vi "Kikusui PLZ-Query Error.vi"(8 "error in":errorcluster, 11 "Kikusui PLZ Setting In":T1={"VISA Resource Name"="", "Baud Rate"=19200, "Stop Bits"=20, "Wait For Read(ms)"=0} {"Stop Bits" items=["1.0"=10, "2.0"=20]; "Baud Rate" items=["2400"=2400, "4800"=4800, "9600"=9600, "19200"=19200]}) -> (0 "error out":errorcluster, 3 "Kikusui PLZ Setting Out":T1={"VISA Resource Name"="", "Baud Rate"=19200, "Stop Bits"=20, "Wait For Read(ms)"=0} {"Stop Bits" items=["1.0"=10, "2.0"=20]; "Baud Rate" items=["2400"=2400, "4800"=4800, "9600"=9600, "19200"=19200]})   [LabVIEW 2018]
uses:
  Data Def/Kikusui PLZ-Setting.ctl
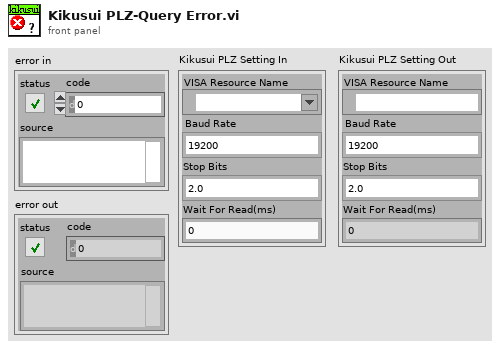
[diagram p1: front panel]
types:
  T1 = typedef "Kikusui PLZ-Setting.ctl" = cluster{"VISA Resource Name":refnum<visa-resource-name>, "Baud Rate":u32, "Stop Bits":u16, "Wait For Read(ms)":u32}
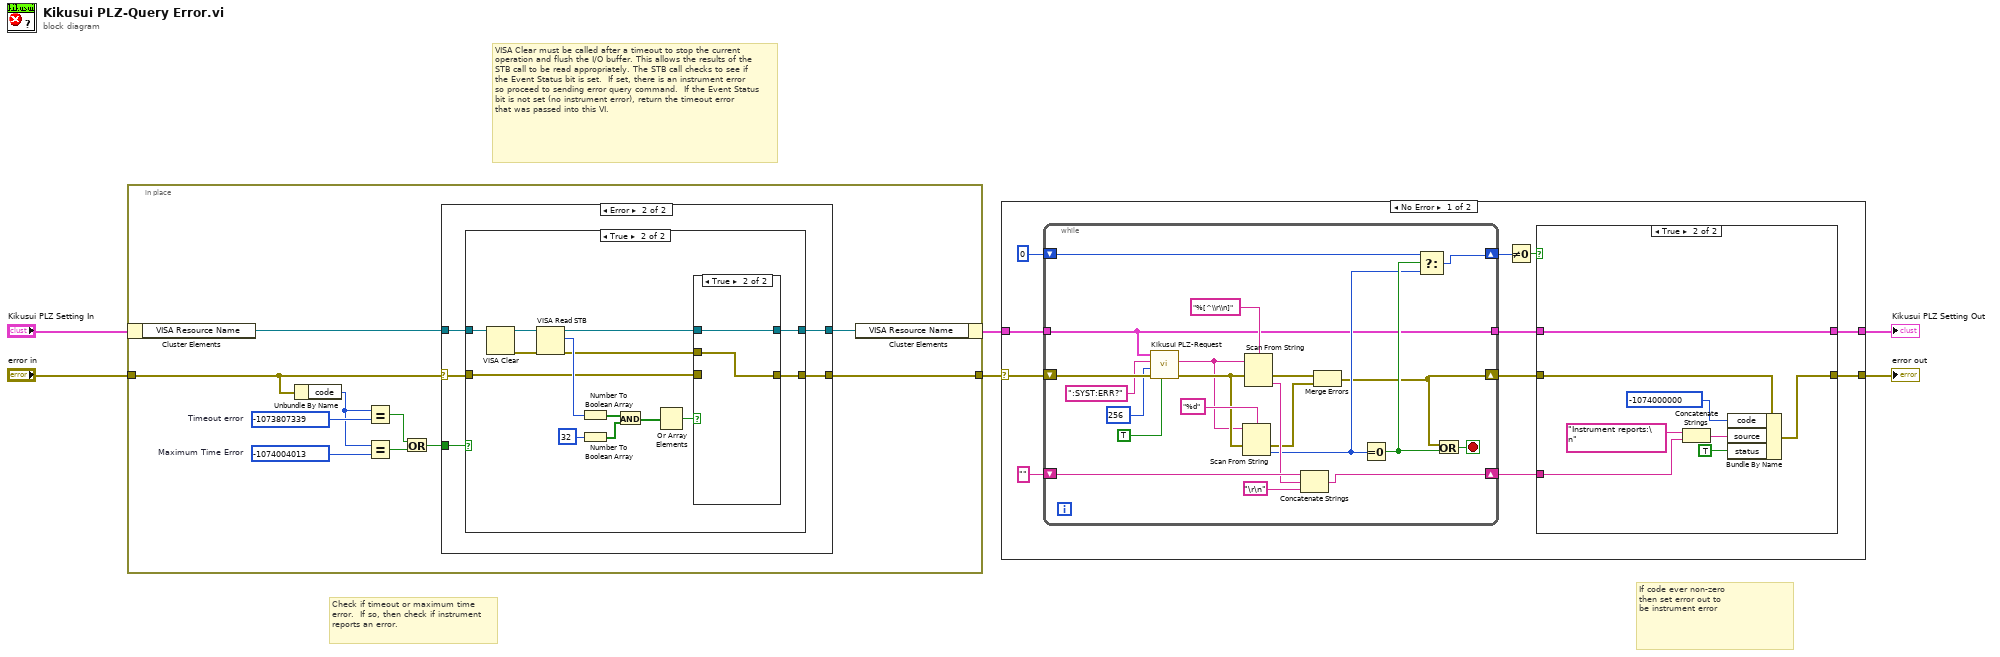
[diagram p0: block diagram]
diagram:
  # "If code ever non-zero\nthen set error out to\nbe instrument error"
  # "Check if timeout or maximum time error.  If so, then check if instrument reports an error."
  # "VISA Clear must be called after a timeout to stop the current operation and flush the I/O buffer. This allows the results of the  STB call to be read appropriately. The STB call checks to see if the Event Status bit is set.  If set, there is an instrument error so proceed to sending error query command.  If the Event Status bit is not set (no instrument error), return the timeout error that was passed into this VI."
  n1 = in-place {
    in-place-border: "error in" -> [w16]
    in-place-border: [w15] -> w4
    w12 = -1074004013  # Maximum Time Error
    w14 = -1073807339  # Timeout error
    n2 = in-place-cluster #1("Kikusui PLZ Setting In") -> ("VISA Resource Name"=w8:refnum<visa-resource-name>)
    n3 = Unbundle By Name(w16) -> ("code"=w13:i32)
    n4 = Equal?(x=w13, y=w14) -> (x = y?=w10:bool)
    n5 = Equal?(x=w13, y=w12) -> (x = y?=w11:bool)
    n6 = Or(x=w10, y=w11) -> (x .or. y?=w9:bool)
    n7 = case shown="Error" w16 {
      selector: w16 -> [w17 w21]
      tunnel: w8 -> [w18 w23]
      tunnel: [w18 w22] -> w7
      tunnel: [w17 w20] -> w15
      tunnel: w9 -> [_ w19]
      frame No Error {
      }
      frame Error {
        n8 = case shown="True" w19 {
          tunnel: w23 -> [w25 w36]
          tunnel: [w25 w26] -> w22
          tunnel: w21 -> [w24 w30]
          tunnel: [w24 w28] -> w20
          frame False {
            # "Error code not a timeout, so best to pass on to user."
          }
          frame True {
            n9 = VISA Clear(VISA resource name=w36) -> (VISA resource name out=w35:refnum<visa-resource-name>, error out=w34:errorcluster)  [unwired: 1 in]
            n10 = VISA Read STB(8:w34, 11:w35) -> (0:w29:errorcluster, 2:w33:u16, 3:w27:refnum<visa-resource-name>)
            n11 = Number To Boolean Array(number=w33) -> (Boolean array=w37:bool[])
            n12 = Number To Boolean Array(number=32) -> (Boolean array=w38:bool[])
            n13 = And(x=w37, y=w38) -> (x .and. y?=w32:bool[])
            n14 = Or Array Elements(Boolean array=w32) -> (logical OR=w31:bool)
            n15 = case shown="True" w31 {
              tunnel: w30 -> [w41 _]
              tunnel: w29 -> [_ w43]
              tunnel: [w41 w43] -> w28
              tunnel: w27 -> [w40 w42]
              tunnel: [w40 w42] -> w26
              frame False {
              }
              frame True {
              }
            }
          }
        }
      }
    }
    n16 = in-place-cluster #1("VISA Resource Name"=w7) -> (w2:T1)
  }
  n17 = case shown="No Error" w4 {
    selector: w4 -> [w48 w86]
    tunnel: [w45 w87] -> w1
    tunnel: w2 -> [w54 w87]
    tunnel: [w44 w86] -> w5
    frame No Error {
      n18 = while {
        tunnel: [w69] -> w46
        tunnel: w54 -> [w69]
        shift-right: [w79] -> w50
        shift-left: "" -> [w82]
        shift-right: [w77] -> w51
        shift-left: 0 -> [w78]
        shift-right: [w72] -> w49
        shift-left: w48 -> [w71]
        stop <- w84 stop-if-true
        n19 = call "Kikusui PLZ-Request.vi"("Response?"=TRUE, "error in"=w71, "byte count"=u32 256, "Command"=":SYST:ERR?" ("Error Query Command"), "Kikusui PLZ Setting In"=w69) -> ("error out"=w68:errorcluster, "Response"=w67:string)  [unwired: 4 in, 1 out]
        n20 = Scan From String(format string="%d", input string=w67, error in=w68) -> (error out=w73:errorcluster, output 1=w75:i32)  [unwired: 2 in, 2 out]
        n21 = Scan From String(format string="%[^\\r\\n]", input string=w67, error in=w68) -> (error out=w74:errorcluster, output 1=w80:string)  [unwired: 2 in, 2 out]
        n22 = Concatenate Strings(w82, w80, "\r\n") -> (w79:string)
        n23 = Merge Errors(w74, w73) -> (w72:errorcluster)
        n24 = Equal To 0?(x=w75) -> (x = 0?=w76:bool)
        n25 = Select(t=w78, s=w76, f=w75) -> (s? t:f=w77:i32)
        n26 = Or(x=w72, y=w76) -> (x .or. y?=w84:bool)
      }
      n27 = Not Equal To 0?(x=w51) -> (x != 0?=w52:bool)
      n28 = case shown="True" w52 {
        tunnel: w50 -> [_ w63]
        tunnel: [w56 w57] -> w44
        tunnel: w49 -> [w56 w61]
        tunnel: w46 -> [w55 w62]
        tunnel: [w55 w62] -> w45
        frame False {
        }
        frame True {
          n29 = Concatenate Strings("Instrument reports:\n" ("Source"), w63) -> (w60:string)
          n30 = Bundle By Name(cluster=w61, "code"=-1074000000 ("Code"), "source"=w60, "status"=TRUE) -> (w57:errorcluster)
        }
      }
    }
    frame Error {
    }
  }
  "error out" <- w5
  "Kikusui PLZ Setting Out" <- w1
